vi "HMF2500 Config Panel.vi"(8 "error in":errorcluster, 11 "session in":T1={"Baud Rate"=9600, "Parity"=0, "Data Bits"=8, "Flow Control"=0} {"Flow Control" items=["None", "XON/XOFF", "RTS/CTS", "XON/XOFF & RTS/CTS", "DTR/DSR", "XON/XOFF & DTR/DSR"]; "Data Bits" items=["7"=7, "8"=8]; "Parity" items=["None", "Odd", "Even", "Mark", "Space"]; "Baud Rate" items=["300"=300, "600"=600, "1200"=1200, "2400"=2400, "4800"=4800, "9600"=9600, "19200"=19200]}) -> (0 "error out":errorcluster, 3 "session out":T1={"Baud Rate"=9600, "Parity"=0, "Data Bits"=8, "Flow Control"=0} {"Flow Control" items=["None", "XON/XOFF", "RTS/CTS", "XON/XOFF & RTS/CTS", "DTR/DSR", "XON/XOFF & DTR/DSR"]; "Data Bits" items=["7"=7, "8"=8]; "Parity" items=["None", "Odd", "Even", "Mark", "Space"]; "Baud Rate" items=["300"=300, "600"=600, "1200"=1200, "2400"=2400, "4800"=4800, "9600"=9600, "19200"=19200]})   [LabVIEW 2020, in "AWG.lvlib"]
doc: "R&S HMF2500 series configuration panel."
uses:
  AWG.lvlib
  HMF2500 Config.ctl
panel:
  in  "btn default":bool
  in  "Data Bits":u16(ring)=8 items=["7"=7, "8"=8]
  in  "Parity":u16(ring) items=["None", "Odd", "Even", "Mark", "Space"]
  in  "Flow Control":u16(ring) items=["None", "XON/XOFF", "RTS/CTS", "XON/XOFF & RTS/CTS", "DTR/DSR", "XON/XOFF & DTR/DSR"]
  in  "Baud Rate":u32
  in  "btn ok":bool
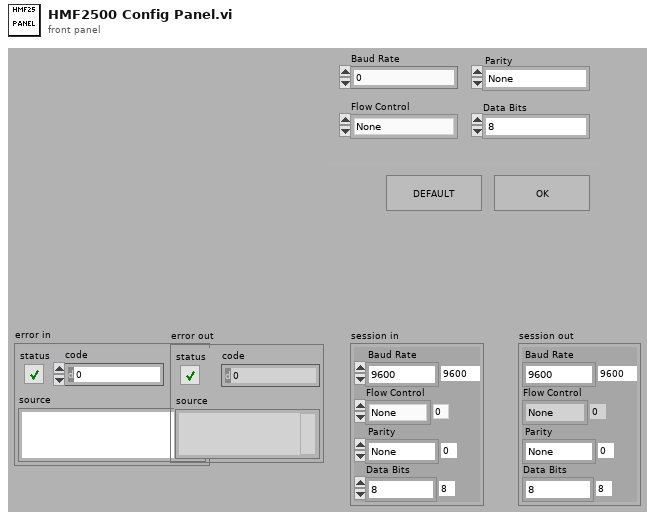
[diagram p1: front panel]
types:
  T1 = typedef "AWG.lvlib/HMF2500 Config.ctl" = cluster{"Baud Rate":u32, "Parity":u16, "Data Bits":u16, "Flow Control":u16}
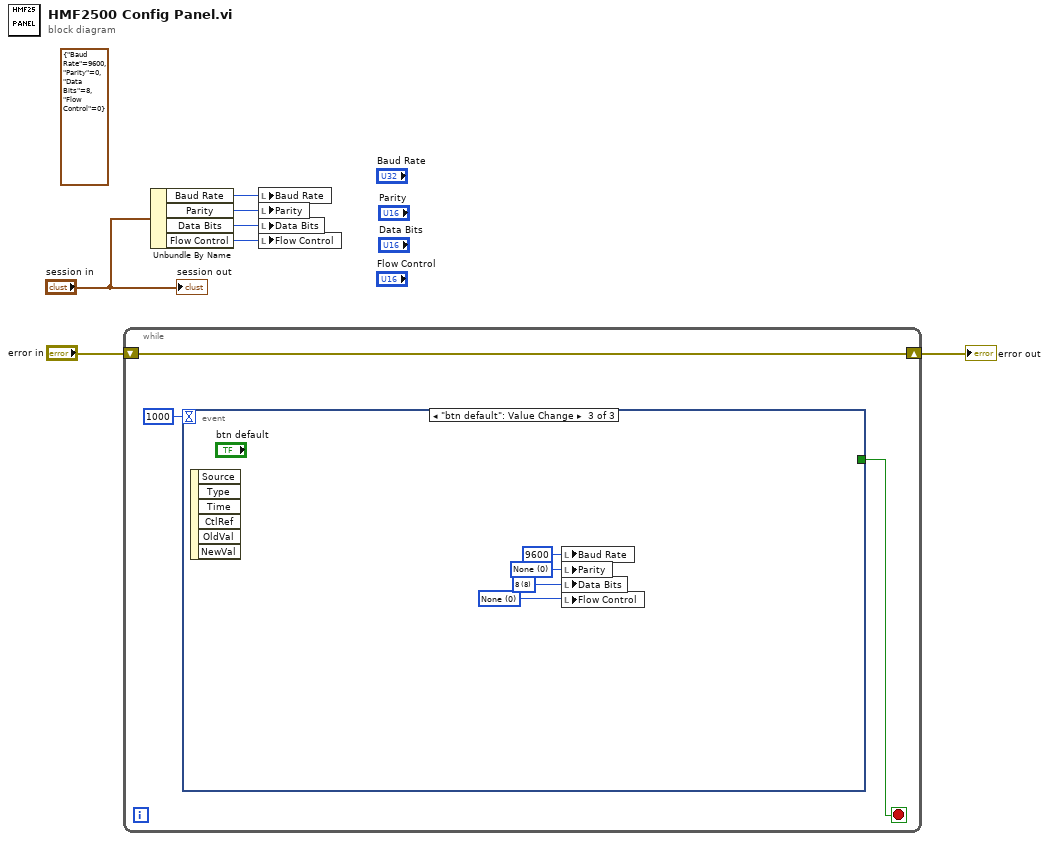
[diagram p0: block diagram]
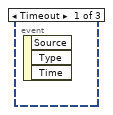
[diagram p2: hidden frame]
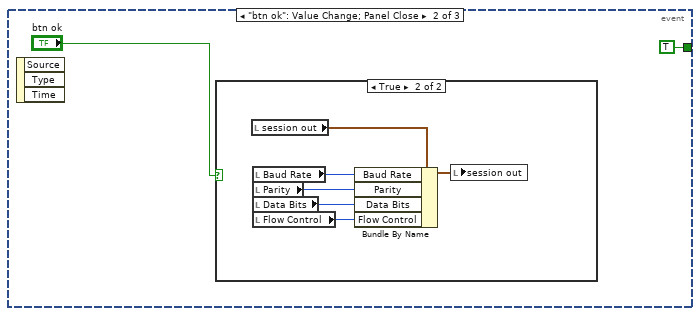
[diagram p3: hidden frame]
diagram:
  (unwired) T1 {"Baud Rate"=9600, "Parity"=0, "Data Bits"=8, "Flow Control"=0} ("session in")
  n1 = while {
    shift-right: [w9] -> w7
    shift-left: "error in" -> [w9]
    stop <- w10 stop-if-true
    n2 = event shown="[2] \"btn default\": Value Change" {
      selector: _ -> [_ _ _]
      dyn-events: _ -> [_ _ _]
      timeout: 1000 -> [_ _ _]
      tunnel: [_ TRUE _] -> w10
      event Timeout {
        n3 = event-data() -> ()  [unwired: 1 in, 3 out]
      }
      event "btn ok": Value Change; Panel Close {
        n4 = event-data() -> ()  [unwired: 1 in, 3 out]
        n5 = case shown="True" "btn ok" {
          frame False {
          }
          frame True {
            n6 = local read "session out"() -> (w17:T1)
            n7 = local read "Baud Rate"() -> (w16:u32)
            n8 = local read "Parity"() -> (w15:u16)
            n9 = local read "Data Bits"() -> (w14:u16)
            n10 = local read "Flow Control"() -> (w13:u16)
            n11 = Bundle By Name(cluster=w17, "Baud Rate"=w16, "Parity"=w15, "Data Bits"=w14, "Flow Control"=w13) -> (w18:T1)
            n12 = local write "session out"(w18) -> ()
          }
        }
      }
      event "btn default": Value Change {
        w19 = u16 0 items=["None", "XON/XOFF", "RTS/CTS", "XON/XOFF & RTS/CTS", "DTR/DSR", "XON/XOFF & DTR/DSR"] ("Flow Control")
        w20 = u16 8 items=["7"=7, "8"=8] ("Data Bits")
        w21 = u16 0 items=["None", "Odd", "Even", "Mark", "Space"] ("Parity")
        n13 = event-data() -> ()  [unwired: 1 in, 6 out]
        n14 = local write "Baud Rate"(u32 9600 ("Baud Rate")) -> ()
        n15 = local write "Parity"(w21) -> ()
        n16 = local write "Data Bits"(w20) -> ()
        n17 = local write "Flow Control"(w19) -> ()
      }
    }
  }
  "error out" <- w7
  n18 = Unbundle By Name("session in") -> ("Baud Rate"=w4:u32, "Parity"=w3:u16, "Data Bits"=w2:u16, "Flow Control"=w1:u16)
  n19 = local write "Baud Rate"(w4) -> ()
  n20 = local write "Parity"(w3) -> ()
  n21 = local write "Data Bits"(w2) -> ()
  n22 = local write "Flow Control"(w1) -> ()
  "session out" <- "session in"
